vi "getData.vi"(8 "error in (no error)":errorcluster, 11 "Instrument.VSource in":refnum<class "Instrument.VNA.lvclass">) -> (0 "error out":errorcluster, 2 "Data":variant, 3 "Instrument.VSource out":refnum<class "Instrument.VNA.lvclass">)   [LabVIEW 2019, in "Instrument.VNA.lvclass"]
uses:
  Instrument.VNA.lvclass
  Typedefs/VNA.Commands--Enum.ctl
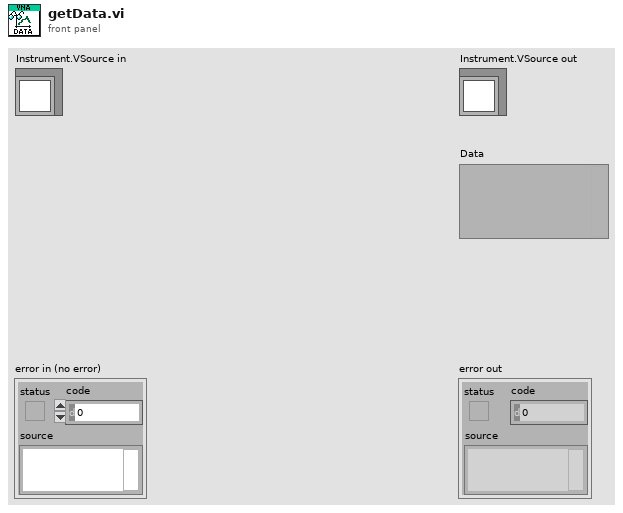
[diagram p1: front panel]
types:
  T1 = typedef "Instrument.VNA.lvclass/VNA.Commands--Enum.ctl" = enum16{"getData", "setAverage", "setFormat", "setMeasurement", "setPower", "setSweep"}
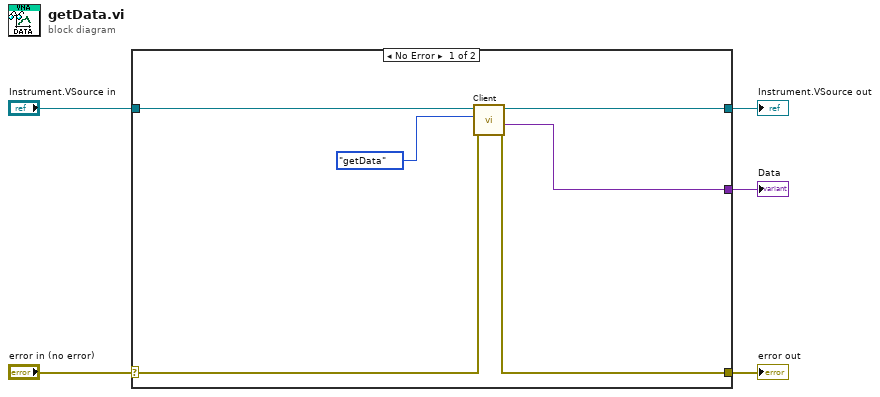
[diagram p0: block diagram]
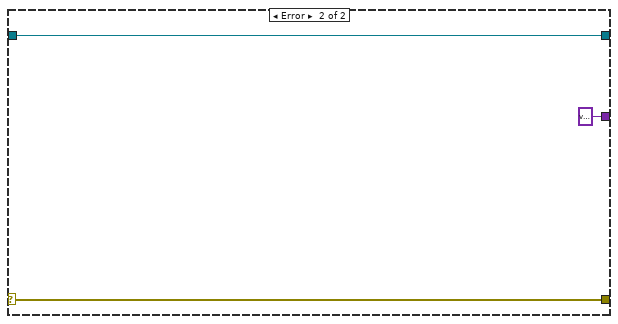
[diagram p2: hidden frame]
diagram:
  n1 = case shown="No Error" "error in (no error)" {
    selector: "error in (no error)" -> [w9 w14]
    tunnel: [w7 w14] -> w4
    tunnel: [w11 w13] -> w2
    tunnel: "Instrument.VSource in" -> [w8 w13]
    tunnel: [w6 variant ("Data out")] -> w1
    frame No Error {
      n2 = call-dynamic "Client.vi"("error in (no error)"=w9, "Command in"=VNA.Commands--Enum."getData" ("Commands"), "Instrument in"=w8) -> ("error out"=w7:errorcluster, "Data out"=w6:variant, "Instrument out"=w11:refnum<class "Instrument.VNA.lvclass">)  [unwired: 5 in, 1 out]
    }
    frame Error {
    }
  }
  "error out" <- w4
  "Instrument.VSource out" <- w2
  "Data" <- w1
